vi "Finish Read.vi"(8 "error in (no error)":errorcluster, 11 "WebsocketStream in":refnum<class "WebsocketStream.lvclass">) -> (0 "error out":errorcluster, 1 "Data":string, 3 "WebsocketStream out":refnum<class "WebsocketStream.lvclass">)   [LabVIEW 2020, in "Stream-Websocket.lvlib" / "WebsocketStream.lvclass"]
uses:
  WebsocketStream.lvclass
  WebsocketStream.lvclass/WebsocketStream.ctl
  OpCode.ctl
  Stream-Websocket.lvlib
  Message Frame.ctl
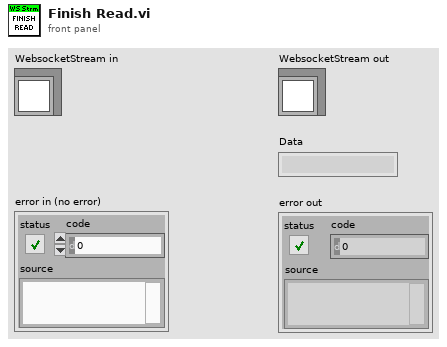
[diagram p1: front panel]
types:
  T1 = typedef "Stream-Websocket.lvlib/Message Frame.ctl" = cluster{"FIN":bool, "RSV1":bool, "RSV2":bool, "RSV3":bool, "MASK":bool, "OpCode":T2, "Length":u64, "MaskingKey":u8[], "Payload":string}
  T2 = typedef "Stream-Websocket.lvlib/OpCode.ctl" = enum8{"Continuation", "Text", "Binary", "Reserved3", "Reserved4", "Reserved5", "Reserved6", "Reserved7", "Close", "Ping", "Pong", "ReservedB", "ReservedC", "ReservedD", "ReservedE", "ReservedF"}
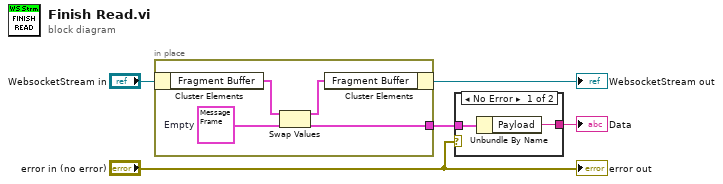
[diagram p0: block diagram]
diagram:
  n1 = in-place {
    in-place-border: [w6] -> w3
    w8 = T1 {"FIN"=FALSE, "RSV1"=FALSE, "RSV2"=FALSE, "RSV3"=FALSE, "MASK"=FALSE, "OpCode"=enum."Continuation", "Length"=0, "MaskingKey"=[], "Payload"=""}  # Empty
    n2 = in-place-cluster #1("WebsocketStream in") -> ("Fragment Buffer"=w9:T1)
    n3 = Swap Values(12:w9, 14:w8) -> (1:w7:T1, 3:w6:T1)  [unwired: 1 in]
    n4 = in-place-cluster #1("Fragment Buffer"=w7) -> (→"WebsocketStream out":refnum<class "WebsocketStream.lvclass">)
  }
  n5 = case shown="No Error" "error in (no error)" {
    tunnel: w3 -> [w11 _]
    tunnel: [w10 _] -> w2
    frame No Error {
      n6 = Unbundle By Name(w11) -> ("Payload"=w10:string)
    }
    frame Error {
    }
  }
  "Data" <- w2
  "error out" <- "error in (no error)"
